vi "getErrorColor.vi"(7 "Criticity":T1, 8 "error in (no error)":errorcluster) -> (0 "error out":errorcluster, 2 "errorColor":u32(colorbox))   [LabVIEW 2013]
uses:
  030 - EVENTS/03 - ToMessageHandlerProcess/enumMessageCriticity.ctl
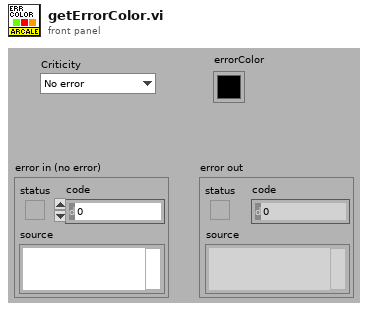
[diagram p1: front panel]
types:
  T1 = typedef "enumMessageCriticity.ctl" = enum16{"No error", "Info", "Warning", "Error", "Fatal error"}
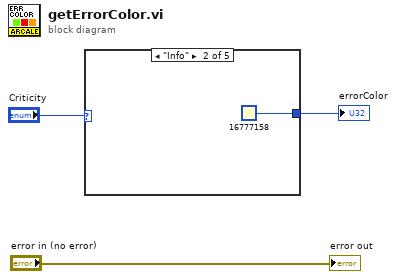
[diagram p0: block diagram]
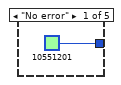
[diagram p2: hidden frame]
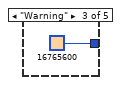
[diagram p3: hidden frame]
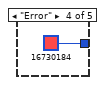
[diagram p4: hidden frame]
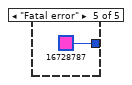
[diagram p5: hidden frame]
diagram:
  n1 = case shown="\"Info\"" "Criticity" {
    tunnel: [u32 10551201 ("errorColor 2") u32 16777158 ("errorColor 2") u32 16765600 ("errorColor 2") u32 16730184 ("errorColor 2") u32 16728787 ("errorColor 2")] -> w2
    frame "No error" {
    }
    frame "Info" {
    }
    frame "Warning" {
    }
    frame "Error" {
    }
    frame "Fatal error" {
    }
  }
  "errorColor" <- w2
  "error out" <- "error in (no error)"
